vi "Write.vi"(4 "File Extension":string="csv", 5 "Maximum File Size (Bytes)":i64, 6 "Enable Calendar Tree":bool=TRUE, 7 "Maximum File Count":i32, 8 "Error In":errorcluster, 9 "Messages":T1[](array[typedef]), 10 "Bulk CSV Buffer In":string, 11 "Log In":refnum<file>) -> (0 "Error Out":errorcluster, 2 "Bulk CSV Buffer Out":string, 3 "Log Out":refnum<file>)   [LabVIEW 2017, in "Toolkit.lvlib" / "File.lvlib"]
uses:
  File.lvlib
  Controls/Statement.ctl
  Controls/Tag.ctl
  Create ISO 8601 File Name.vi
  Write Header.vi
  Create Calendar Folder Tree.vi
  Get Oldest File.vi
  <vilib>/Utility/libraryn.llb/Check if File or Folder Exists.vi
  Toolkit.lvlib
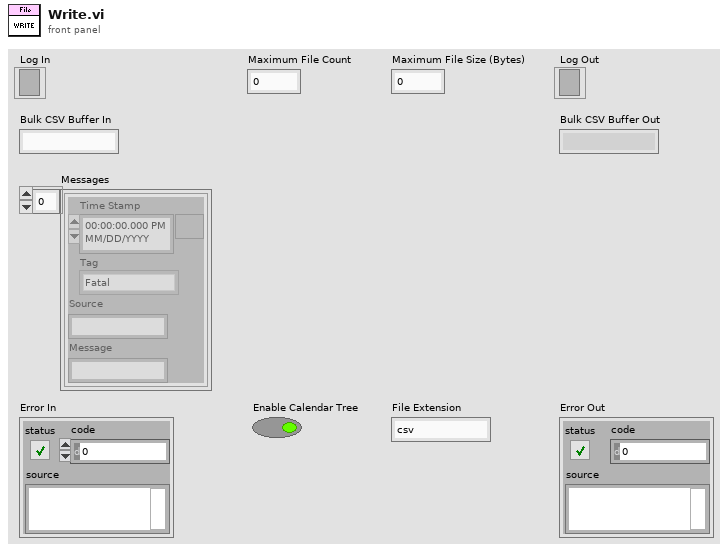
[diagram p1: front panel]
types:
  T1 = typedef "Toolkit.lvlib/Statement.ctl" = cluster{"Time Stamp":timestamp, "Tag":T2, "Source":string, "Message":string}
  T2 = typedef "Toolkit.lvlib/Tag.ctl" = enum16{"Fatal", "Error", "Warn", "Info", "Debug", "Trace"}
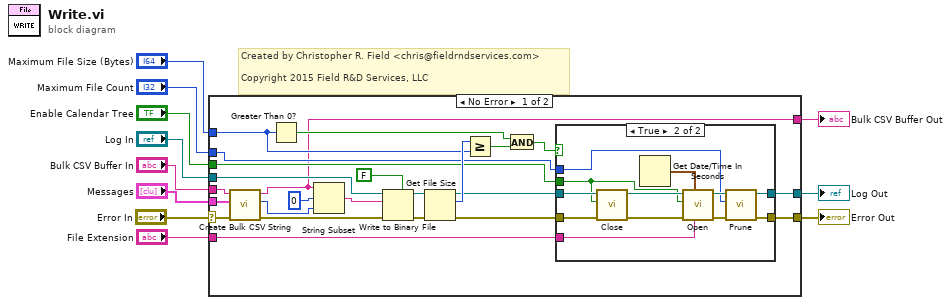
[diagram p0: block diagram]
diagram:
  # "Created by Christopher R. Field <chris@fieldrndservices.com>\n\nCopyright 2015 Field R&D Services, LLC"
  n1 = case shown="No Error" "Error In" {
    selector: "Error In" -> [w19 w51]
    tunnel: "Log In" -> [w35 w52]
    tunnel: "Messages" -> [w17 _]
    tunnel: [w25 w52] -> w8
    tunnel: [w24 w51] -> w7
    tunnel: "Maximum File Size (Bytes)" -> [w26 _]
    tunnel: "Enable Calendar Tree" -> [w23 _]
    tunnel: "Maximum File Count" -> [w22 _]
    tunnel: "File Extension" -> [w21 _]
    tunnel: "Bulk CSV Buffer In" -> [w16 w50]
    tunnel: [w12 w50] -> w1
    frame No Error {
      n2 = call "Create Bulk CSV String.vi"("Error In"=w19, "Messages"=w17, "Bulk CSV Buffer In"=w16) -> ("Error Out"=w18:errorcluster, "CSV Length"=w15:i32, "Bulk CSV Buffer Out"=w12:string)  [unwired: 6 in]
      n3 = Greater Than 0?(x=w26) -> (x > 0?=w33:bool)
      n4 = String Subset(string=w12, offset (0)=0, length (rest)=w15) -> (substring=w13:string)
      n5 = Write to Binary File(file (use dialog)=w35, data=w13, error in=w18, 5:FALSE ("prepend array or string size? (T)")) -> (refnum out=w28:refnum<file>, error out=w27:errorcluster)  [unwired: 2 in, 1 out]
      n6 = Get File Size(file=w28, error in=w27) -> (refnum out=w30:refnum<file>, size (in bytes)=w32:i64, 0:w29:errorcluster)
      n7 = Greater Or Equal?(x=w32, y=w26) -> (x >= y?=w34:bool)
      n8 = And(x=w33, y=w34) -> (x .and. y?=w31:bool)
      n9 = case shown="True" w31 {
        tunnel: [w37 w41] -> w25
        tunnel: [w36 w42] -> w24
        tunnel: w30 -> [w37 w48]
        tunnel: w29 -> [w36 w47]
        tunnel: w23 -> [_ w39]
        tunnel: w22 -> [_ w40]
        tunnel: w21 -> [_ w38]
        frame False {
        }
        frame True {
          n10 = call "Close.vi"("Error In"=w47, "Enable Calendar Tree"=w39, "Log In"=w48) -> ("Error Out"=w46:errorcluster, "Base Log Folder"=w45:path)  [unwired: 7 in]
          n11 = Get Date/Time In Seconds() -> (seconds since 1Jan1904=w49:timestamp)
          n12 = call "Open.vi"("File Extension"=w38, "Start Time Stamp"=w49, "Error In"=w46, "Enable Calendar Tree"=w39, "Base Folder"=w45) -> ("Error Out"=w43:errorcluster, "Log Out"=w44:refnum<file>)  [unwired: 5 in]
          n13 = call "Prune.vi"("Error In"=w43, "Maximum File Count"=w40, "File In"=w44) -> ("Error Out"=w42:errorcluster, "File Out"=w41:refnum<file>)  [unwired: 7 in]
        }
      }
    }
    frame Error {
    }
  }
  "Log Out" <- w8
  "Error Out" <- w7
  "Bulk CSV Buffer Out" <- w1
